vi "Main.vi"   [LabVIEW 2018, in "FacadePatternDemo.lvclass"]
uses:
  FacadePatternDemo.lvclass
  VideoConversionFacade Class/VideoConversionFacade.lvclass
  ConsoleOut/Print Options.ctl
types:
  T1 = typedef "Print Options.ctl" = enum16{"Create", "Get Reference", "Print", "Print Header", "Close"}
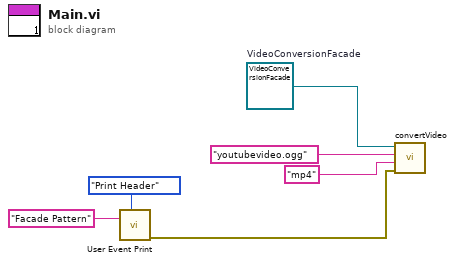
[diagram p0: block diagram]
diagram:
  w6 = refnum<class "VideoConversionFacade.lvclass"> refnum  # VideoConversionFacade
  n1 = call "User Event Print.vi"("Options"=Print_Options."Print Header", "String to Print"="Facade Pattern") -> ("error out"=w3:errorcluster)  [unwired: 8 in, 1 out]
  n2 = call "convertVideo.vi"("error in (no error)"=w3, "format"="mp4", "fileName"="youtubevideo.ogg", "VideoConversionFacade in"=w6) -> ()  [unwired: 5 in, 3 out]
